vi "BreakfastMenu_Create.vi"(8 "Error In":errorcluster, 11 "reference in":refnum<class "BreakfastMenu.lvclass">) -> (0 "Error Out":errorcluster, 3 "reference out":refnum<class "BreakfastMenu.lvclass">)   [LabVIEW 2020, in "BreakfastMenu.lvclass"]
uses:
  BreakfastMenu.lvclass
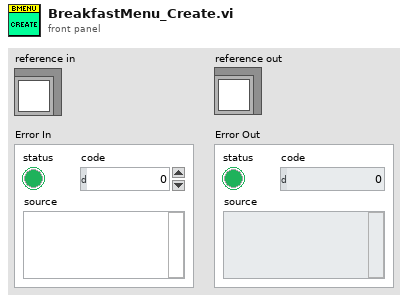
[diagram p1: front panel]
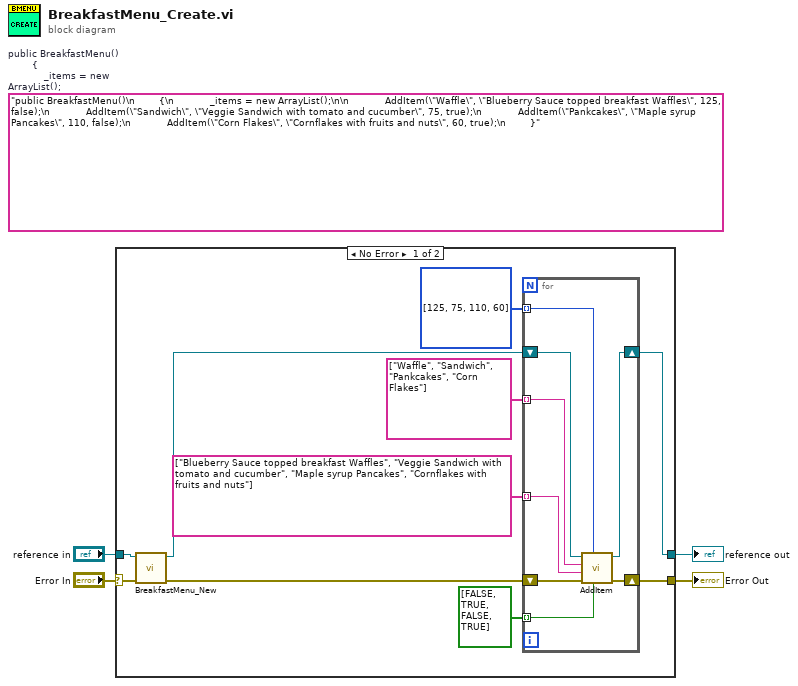
[diagram p0: block diagram]
diagram:
  (unwired) "public BreakfastMenu()\n        {\n            _items = new ArrayList();\n\n            AddItem(\"Waffle\", \"Blueberry Sauce topped breakfast Waffles\", 125, false);\n            AddItem(\"Sandwich\", \"Veggie Sandwich with tomato and cucumber\", 75, true);\n            AddItem(\"Pankcakes\", \"Maple syrup Pancakes\", 110, false);\n            AddItem(\"Corn Flakes\", \"Cornflakes with fruits and nuts\", 60, true);\n        }"  # public BreakfastMenu()         {             _items = new ArrayList();              AddItem("Waffle", "Blueberry Sauce topped breakfast Waffles", 125, false);             AddItem("Sandwich", "Veggie Sandwich with tomato and cucumber", 75, true);             AddItem("Pankcakes", "Maple syrup Pancakes", 110, false);             AddItem("Corn Flakes", "Cornflakes with fruits and nuts", 60, true);         }
  n1 = case shown="No Error" "Error In" {
    selector: "Error In" -> [w13 w24]
    tunnel: [w9 w24] -> w3
    tunnel: "reference in" -> [w14 w23]
    tunnel: [w10 w23] -> w1
    frame No Error {
      n2 = call "BreakfastMenu_New.vi"("error in (no error)"=w13, "reference in"=w14) -> ("error out"=w11:errorcluster, "reference out"=w12:refnum<class "BreakfastMenu.lvclass">)  [unwired: 6 in, 2 out]
      n3 = for {
        shift-right: [w20] -> w10
        shift-left: w12 -> [w22]
        shift-right: [w19] -> w9
        shift-left: w11 -> [w21]
        tunnel: string[] ["Waffle", "Sandwich", "Pankcakes", "Corn Flakes"] -> [w18] mode=indexing
        tunnel: string[] ["Blueberry Sauce topped breakfast Waffles", "Veggie Sandwich with tomato and cucumber", "Maple syrup Pancakes", "Cornflakes with fruits and nuts"] -> [w17] mode=indexing
        tunnel: i32[] [125, 75, 110, 60] ("Price") -> [w16] mode=indexing
        tunnel: bool[] [FALSE, TRUE, FALSE, TRUE] ("Veg") -> [w15] mode=indexing
        n4 = call "AddItem.vi"("Veg"=w15, "Price"=w16, "Error In"=w21, "Description"=w17, "Name"=w18, "reference in"=w22) -> ("Error Out"=w19:errorcluster, "reference out"=w20:refnum<class "BreakfastMenu.lvclass">)  [unwired: 4 in]
      }
    }
    frame Error {
      # "VI-TechBaseTemplate_Simple_4x4x4"
    }
  }
  "Error Out" <- w3
  "reference out" <- w1
